vi "createInterface.vi"(8 "error in (no error)":errorcluster, 11 "OrionBMS in":refnum<class "OrionBMSClass.lvclass">) -> (0 "error out":errorcluster, 2 "interface object out":refnum<k20>, 3 "OrionBMS out":refnum<class "OrionBMSClass.lvclass">)   [LabVIEW 2018, in "OrionBMSClass.lvclass"]
uses:
  OrionBMSClass.lvclass
  <vilib>/CANopenLib/CANOPEN.llb/CANopen Interface Create.vi
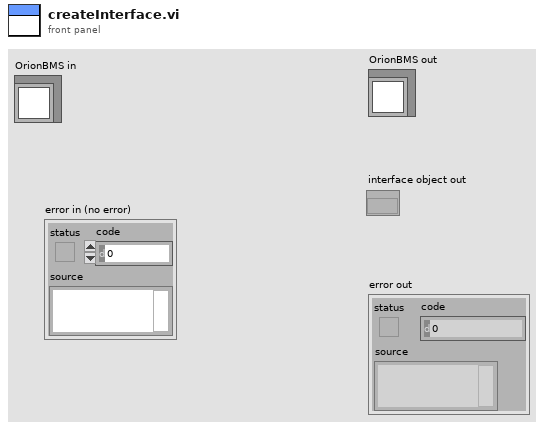
[diagram p1: front panel]
types:
  T1 = enum32{"1 Mbit/s", "800 kbit/s", "500 kbit/s", "250 kbit/s", "125 kbit/s", "50 kbit/s", "20 kbit/s", "10 kbit/s", ""}
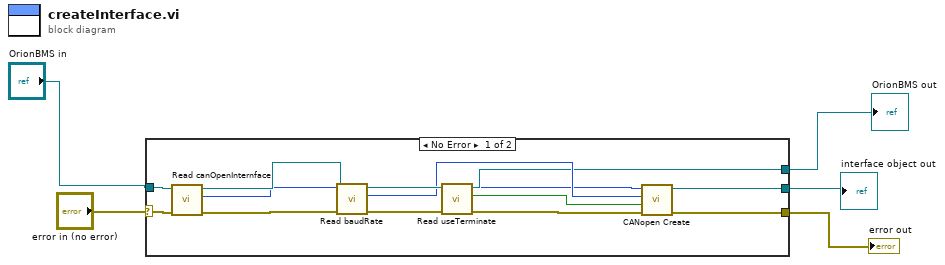
[diagram p0: block diagram]
diagram:
  n1 = case shown="No Error" "error in (no error)" {
    selector: "error in (no error)" -> [w17 w19]
    tunnel: "OrionBMS in" -> [w18 w20]
    tunnel: [w9 _] -> w4
    tunnel: [w7 w20] -> w3
    tunnel: [w8 w19] -> w2
    frame No Error {
      n2 = call-dynamic "Read canOpenInternface.vi"("error in (no error)"=w17, "OrionBMS in"=w18) -> ("error out"=w14:errorcluster, "canOpenInterface"=w6:u32, "OrionBMS out"=w16:refnum<class "OrionBMSClass.lvclass">)  [unwired: 7 in]
      n3 = call "Read baudRate.vi"("error in (no error)"=w14, "OrionBMSClass.lvclass"=w16) -> ("error out"=w13:errorcluster, "baudRate"=w11:T1, "OrionBMSClass.lvclass 2"=w15:refnum<class "OrionBMSClass.lvclass">)  [unwired: 7 in]
      n4 = call-dynamic "Read useTerminate .vi"("error in (no error)"=w13, "OrionBMS in"=w15) -> ("error out"=w10:errorcluster, "useTerminate"=w12:bool, "OrionBMS out"=w7:refnum<class "OrionBMSClass.lvclass">)  [unwired: 7 in]
      n5 = call-poly <vilib>:"CANopen Create.vi"("error in (no error)"=w10, "termination? (F)"=w12, "baud rate"=w11, "interface name"=w6) -> ("error out"=w8:errorcluster, "interface object out"=w9:refnum<k20>)  [unwired: 6 in]
    }
    frame Error {
    }
  }
  "interface object out" <- w4
  "OrionBMS out" <- w3
  "error out" <- w2
